vi "JKI State Machine Helper.vi"(6 "Variant in":variant, 7 "Shift Pressed?":bool, 8 "error in (no error)":errorcluster, 10 "QD Combo Box Ref":refnum<vi>, 11 "QD Launch VI Ref":refnum<vi>) -> (0 "error out":errorcluster, 4 "Variant out":variant)   [LabVIEW 2020]
doc: "Launches JKI State Machine Helper.\n\nDefault Shortcut - [j]"
uses:
  JKI State Machine API/source/JKI SM/JKI SM.lvclass
panel:
  in  "Undo Name":string="Quick Drop Keyboard Shortcut"
  # "Do not change the connector pane of this VI.\n\nSee the block diagram for directions on how to use this template."
  # "Specify the name of the Undo transaction"
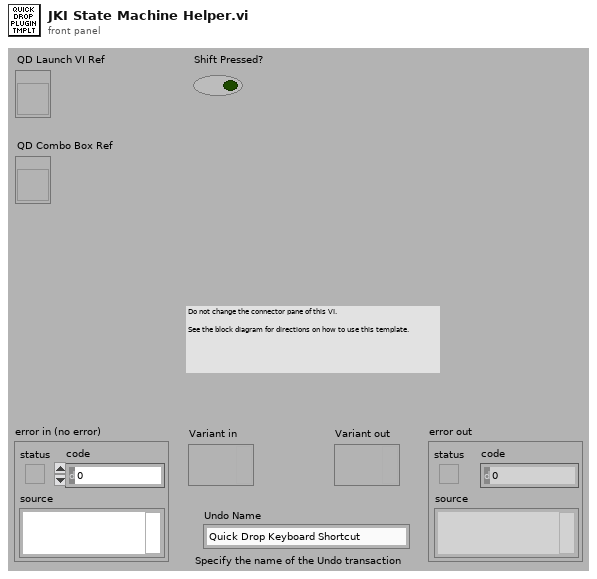
[diagram p1: front panel]
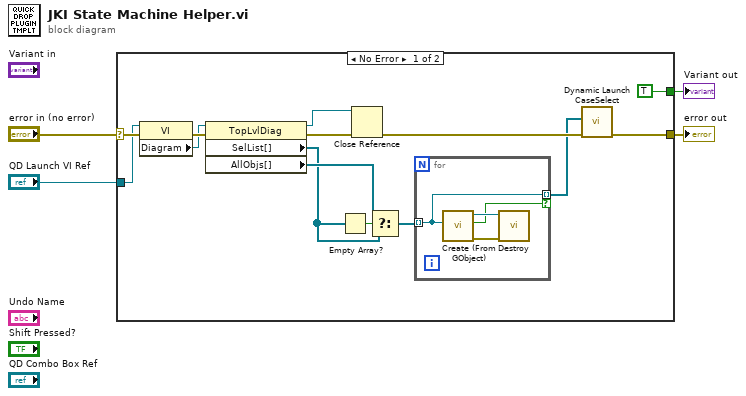
[diagram p0: block diagram]
diagram:
  n1 = case shown="No Error" "error in (no error)" {
    selector: "error in (no error)" -> [w18 w23]
    tunnel: [w10 w23] -> w3
    tunnel: "QD Launch VI Ref" -> [w17 _]
    tunnel: [TRUE _] -> w1
    frame No Error {
      n2 = property class="VI"(reference=w17, error in=w18) -> (error out=w14:errorcluster, "Diagram"=w13:refnum<vi>)  [unwired: 1 out]
      n3 = property class="TopLvlDiag"(reference=w13, error in=w14) -> (reference out=w11:refnum<vi>, error out=w12:errorcluster, "SelList[]"=w6:refnum<vi>[], "AllObjs[]"=w8:refnum<vi>[])
      n4 = Empty Array?(array=w6) -> (empty?=w9:bool)
      n5 = Close Reference(reference=w11, error in (no error)=w12) -> (error out=w15:errorcluster)
      n6 = Select(t=w8, s=w9, f=w6) -> (s? t:f=w7:refnum<vi>[])
      n7 = for {
        tunnel: w7 -> [w19] mode=indexing
        tunnel: [w19] -> w5 mode=indexing if=w20
        n8 = call "Create (From GObject).vi"("GObject"=w19) -> ("error out"=w21:errorcluster, "Found JKI SMs?"=w20:bool, "JKI SM out"=w22:refnum<class "JKI SM.lvclass">)  [unwired: 7 in, 1 out]
        n9 = call "Destroy.vi"("error in (no error)"=w21, "JKI SM in"=w22) -> ()  [unwired: 9 in, 1 out]
      }
      n10 = call "Dynamic Launch CaseSelect.vi"("error in (no error)"=w15, "Active VI Sel. List[]"=w5) -> ("error out"=w10:errorcluster)  [unwired: 9 in]
    }
    frame Error {
    }
  }
  "error out" <- w3
  "Variant out" <- w1
